vi "iso8601_string_to_timestamp.vi"(11 "ISO8601 Timestamp String":string) -> (2 "valid?":bool, 3 "Time Stamp":timestamp format="%<%x %.3X>T")   [LabVIEW 2020, in "Nominal Client.lvclass"]
doc: "Parses an ISO8601 date-time string and converts it into a LabVIEW timestamp."
uses:
  Nominal Client.lvclass
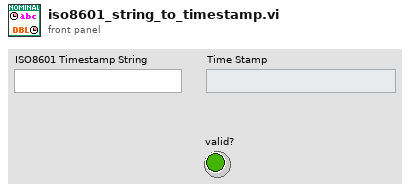
[diagram p1: front panel]
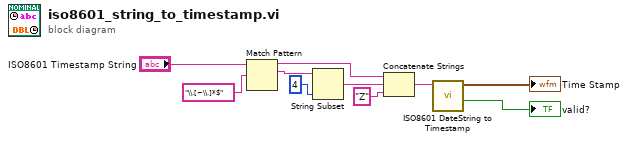
[diagram p0: block diagram]
diagram:
  n1 = Match Pattern(string="ISO8601 Timestamp String", regular expression="\\.[~\\.]*$") -> (before substring=w4:string, match substring=w9:string)  [unwired: 3 out]
  n2 = String Subset(string=w9, length (rest)=4 ("offset (0)")) -> (substring=w8:string)  [unwired: 1 in]
  n3 = Concatenate Strings(w4, w8, "Z" ("string")) -> (w6:string)
  n4 = call <vilib>:"ISO8601 DateString to Timestamp.vi"("ISO8601 String"=w6) -> ("valid?"=→"valid?":bool, "Timestamp"=→"Time Stamp":timestamp)  [unwired: 8 in, 1 out]
